vi "MGI String Pattern Match Exists.vi"(2 "Patterns to Try":string[](array[string]), 3 "String":string) -> (0 "Index of First Pattern Matched":i32, 1 "Match Found":bool)   [LabVIEW 2020]
doc: "Returns true if any of the Patterns to Try are found in String. The patterns are tried in order, and the index of the first pattern to match is returned. If no match is found, the returned index is equal -1. \n\nAuthored by Thomas E. Henage\nsupport@mooregoodideas.com\nwww.mooregoodideas.com\n\nCopyright (c) 2010, Moore Good Ideas, Inc.\n\nAll rights reserved.\n\nRedistribution and use in source and binary forms, with or without modification, are permitted provided that the following conditions are met:\n\n * Redistributions of source code must retain the above copyright notice, this list of conditions and the following disclaimer.\n * Redistributions in binary form must reproduce the above copyright notice, this list of conditions and the following disclaimer in the documentation and/or other materials provided with the distribution.\n * Neither the name of Moore Good Ideas, Inc. nor the names of its contributors may be used to endorse or promote products derived from this software without specific prior written permission.\n\nTHIS SOFTWARE IS PROVIDED BY THE COPYRIGHT HOLDERS AND CONTRIBUTORS \"AS IS\" AND ANY EXPRESS OR IMPLIED WARRANTIES, INCLUDING, BUT NOT LIMITED TO, THE IMPLIED WARRANTIES OF MERCHANTABILITY AND FITNESS FOR A PARTICULAR PURPOSE ARE DISCLAIMED. IN NO EVENT SHALL THE COPYRIGHT OWNER OR CONTRIBUTORS BE LIABLE FOR ANY DIRECT, INDIRECT, INCIDENTAL, SPECIAL, EXEMPLARY, OR CONSEQUENTIAL DAMAGES (INCLUDING, BUT NOT LIMITED TO, PROCUREMENT OF SUBSTITUTE GOODS OR SERVICES; LOSS OF USE, DATA, OR PROFITS; OR BUSINESS INTERRUPTION) HOWEVER CAUSED AND ON ANY THEORY OF LIABILITY, WHETHER IN CONTRACT, STRICT LIABILITY, OR TORT (INCLUDING NEGLIGENCE OR OTHERWISE) ARISING IN ANY WAY OUT OF THE USE OF THIS SOFTWARE, EVEN IF ADVISED OF THE POSSIBILITY OF SUCH DAMAGE."
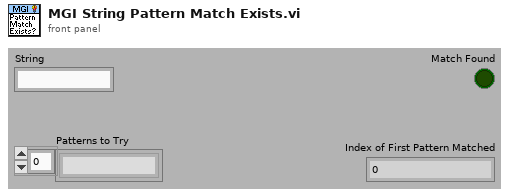
[diagram p1: front panel]
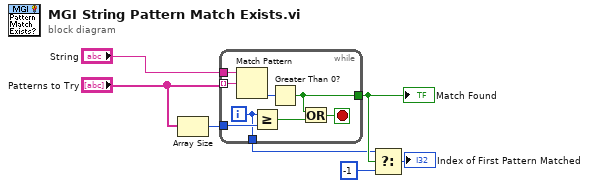
[diagram p0: block diagram]
diagram:
  n1 = Array Size(array="Patterns to Try") -> (size(s)=w7:i32)
  n2 = while {
    tunnel: "String" -> [w15]
    tunnel: "Patterns to Try" -> [w14] mode=indexing
    tunnel: [w11] -> w4
    tunnel: w7 -> [w10]
    tunnel: [w8] -> w3
    i -> [w8]
    stop <- w12 stop-if-true
    n3 = Match Pattern(string=w15, regular expression=w14) -> (offset past match=w13:i32)  [unwired: 4 out]
    n4 = Greater Or Equal?(x=w8, y=w10) -> (x >= y?=w9:bool)
    n5 = Greater Than 0?(x=w13) -> (x > 0?=w11:bool)
    n6 = Or(x=w11, y=w9) -> (x .or. y?=w12:bool)
  }
  "Match Found" <- w4
  n7 = Select(t=w3, s=w4, f=-1) -> (s? t:f=→"Index of First Pattern Matched":i32)
